vi "Cooldown.vi"(8 "error in (no error)":errorcluster, 11 "BaseProducer in":refnum<class "BaseProducer.lvclass">) -> (0 "error out":errorcluster, 2 "Cooldown State":dbl[](array[numeric])=[1.0, 0.0, 0.0, 0.0], 3 "BaseProducer out":refnum<class "BaseProducer.lvclass">)   [LabVIEW 2013, in "BaseProducer.lvclass"]
doc: "This method puts the burner into a cool down state, wherein air is ON, and all fuel mass flow controllers are off."
uses:
  BaseProducer.lvclass
  BaseProducer.lvclass/BaseProducer.ctl
  <vilib>/DAQmx/write.llb/DAQmx Write (Analog 1D DBL NChan 1Samp).vi
  <vilib>/DAQmx/miscellaneous.llb/DAQmx Fill In Error Info.vi
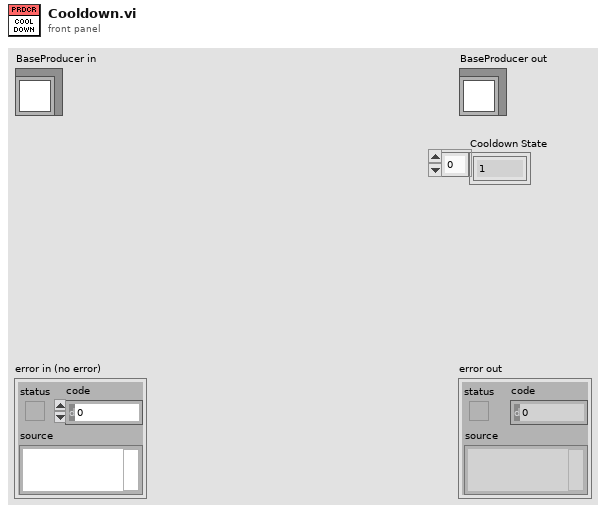
[diagram p1: front panel]
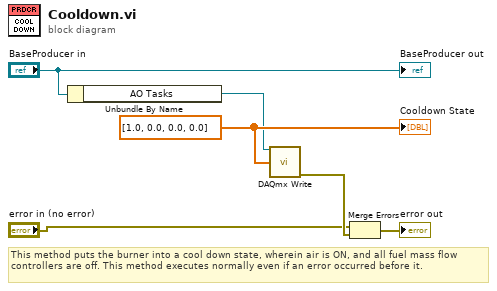
[diagram p0: block diagram]
diagram:
  w5 = dbl[] [1.0, 0.0, 0.0, 0.0]
  # "This method puts the burner into a cool down state, wherein air is ON, and all fuel mass flow controllers are off. This method executes normally even if an error occurred before it."
  n1 = Unbundle By Name("BaseProducer in") -> ("AO Tasks"=w4:refnum<k21>)
  n2 = call-poly <vilib>:"DAQmx Write.vi"("task/channels in"=w4, "data"=w5) -> ("error out"=w2:errorcluster)  [unwired: 11 in, 2 out]
  n3 = Merge Errors("error in (no error)", w2) -> (→"error out":errorcluster)
  "BaseProducer out" <- "BaseProducer in"
  "Cooldown State" <- w5
